vi "Write Hook.vi"(8 "Error In":errorcluster, 10 "Hook":refnum<class "Process.lvclass">, 11 "Conpiler In":refnum<class "Compiler.lvclass">) -> (0 "Error Out":errorcluster, 3 "Compiler Out":refnum<class "Compiler.lvclass">)   [LabVIEW 2018, in "Toolkit.lvlib" / "Compiler.lvclass"]
uses:
  Compiler.lvclass
  Hooks/Compile/Process/Process.lvclass
  Compiler.lvclass/Compiler.ctl
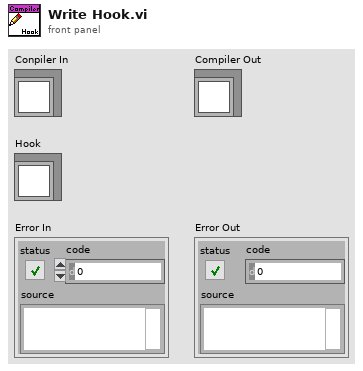
[diagram p1: front panel]
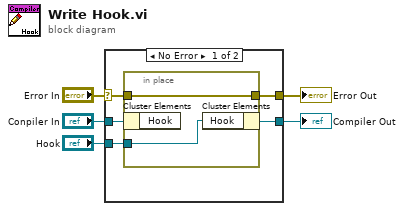
[diagram p0: block diagram]
diagram:
  n1 = case shown="No Error" "Error In" {
    selector: "Error In" -> [w7 w14]
    tunnel: "Conpiler In" -> [w10 w13]
    tunnel: [w6 w14] -> w3
    tunnel: [w9 w13] -> w2
    tunnel: "Hook" -> [w8 _]
    frame No Error {
      n2 = in-place {
        in-place-border: w8 -> [w12]
        in-place-border: w7 -> [w11]
        in-place-border: [w11] -> w6
        n3 = in-place-cluster #1(w10) -> ()  [unwired: 1 out]
        n4 = in-place-cluster #1("Hook"=w12) -> (w9:refnum<class "Compiler.lvclass">)
      }
    }
    frame Error {
    }
  }
  "Error Out" <- w3
  "Compiler Out" <- w2
